vi "S2DS_INSTRUMENTS INVENTORY.vi"(5 "Instrument Info (in)":T2, 6 "Port list (in)":T1, 7 "error in":errorcluster) -> (0 "Instrument info (out)":T2, 1 "Port lists (out)":T1, 2 "OK 2":bool, 3 "Error (out)":errorcluster, 4 "Use array instrument":bool)   [LabVIEW 2025]
uses:
  TYPE DEFS/S2DS_VISA Read.ctl
  INST DRIVERS/My Current source/KE622x -- Output Low Connection.ctl
  INST DRIVERS/My Current source/KE622x -- Current Range.ctl
  INST DRIVERS/My Current source/KE622x -- Current Ranges.ctl
  TYPE DEFS/S2DS_Port lists.ctl
  TYPE DEFS/S2DS_Instrument Info.ctl
  TYPE DEFS/S2DS_Instrument parameters.ctl
  TYPE DEFS/S2DS_External write instrument settings.ctl
  INST DRIVERS/DAQ/MyDaq.lvlib
  INST DRIVERS/Cryo/Cryo.lvlib
  INST DRIVERS/DilutionFridge/MyTriton.lvlib
  INST DRIVERS/MySMU/MySMU.lvlib
  INST DRIVERS/My Current source/My Current Source.lvlib
panel:
  in  "Clear error":bool
  in  "Tab Control":T4(tab)
  in  "DAQ AO Address":tag[](array[tag]) caption="DAQ AO Addresses"
  in  "Min":dbl[](array[numeric])=[-10.0, -10.0, -10.0, -10.0]
  in  "Max":dbl[](array[numeric])=[10.0, 10.0, 10.0, 10.0]
  out "DAQ AO names":string[](array[string])=["DAQ1 AO 0", "DAQ1 AO 1", "DAQ2 AO 0", "DAQ2 AO 1"]
  out "DAQ  AI names":string[](array[string])=["DAQ1 AO 0", "DAQ1 AO 1", "DAQ2 AO 0", "DAQ2 AO 1"]
  in  "DAQ AI address":tag[](array[tag]) caption="DAQ AI Addresses"
  out "Present values":dbl[](array[numeric])
  in  "Use DAQ?":bool
  in  "Use Lock in 4":bool
  in  "Input ports 4":u16(ring) caption="Output ports" items=["None", "Sine out freq, amp", "AUX OUT", "Both Sine out and AUX OUT"]
  in  "Output ports 4":u16(ring) caption="Input ports" items=["X,Y,R,Theta", "Only AUX IN", "X,Y,R,Theta,AUX IN"]
  in  "VISA resource name lock in 4":refnum<visa-resource-name>
  in  "Measuring mode 4":enum16{"Voltage", "Current"}(ring) caption="Measuring mode"
  in  "Measuring mode 1":enum16{"Voltage", "Current"}(ring) caption="Measuring mode"
  in  "Use Lock in 1":bool
  in  "VISA resource name lock in 1":refnum<visa-resource-name>
  in  "Input ports":u16(ring) items=["X,Y,R,Theta", "Only AUX IN", "X,Y,R,Theta,AUX IN"]
  in  "Output ports":u16(ring)=1 items=["None", "Sine out freq, amp", "AUX OUT", "Both Sine out and AUX OUT"]
  in  "Use Lock in 2":bool
  in  "Input ports 2":u16(ring) caption="Output ports" items=["None", "Sine out freq, amp", "AUX OUT", "Both Sine out and AUX OUT"]
  in  "Output ports 2":u16(ring) caption="Input ports" items=["X,Y,R,Theta", "Only AUX IN", "X,Y,R,Theta,AUX IN"]
  in  "VISA resource name lock in 2":refnum<visa-resource-name>
  in  "Use Lock in 3":bool
  in  "Input ports 3":u16(ring) caption="Output ports" items=["None", "Sine out freq, amp", "AUX OUT", "Both Sine out and AUX OUT"]
  in  "Output ports 3":u16(ring) caption="Input ports" items=["X,Y,R,Theta", "Only AUX IN", "X,Y,R,Theta,AUX IN"]
  in  "VISA resource name lock in 3":refnum<visa-resource-name>
  in  "Measuring mode 2":enum16{"Voltage", "Current"}(ring)=enum."Current" caption="Measuring mode"
  in  "Measuring mode 3":enum16{"Voltage", "Current"}(ring) caption="Measuring mode"
  in  "Auto clear error? 2":bool caption="Auto clear error?"
  in  "Precision 2":dbl=0.0001 caption="Precision"
  in  "GPIB address":string="25"
  in  "Use wet cryo magnet?":bool
  in  "Select channel":u16(ring)=8 items=["PT2 Head"=1, "PT2 Plate"=2, "Still Plate"=3, "Cold Plate"=4, "MC Plate Cernox"=5, "PT1 Head"=6, "PT1 Plate"=7, "MC Plate RuO2"=8, "Magnet"=13]
  in  "Use DF?":bool caption="Use  Triton RI?"
  in  "Hold at end?":bool=TRUE
  in  "Precision":dbl=0.001
  in  "Auto clear error?":bool=TRUE
  in  "Initialize magnet?":bool
  in  "Initialize cryo magnet?":bool
  in  "Info magnet":bool
  in  "IP address":string="192.168.0.107"
  in  "Address":refnum<visa-resource-name>
  in  "Write Temp":string(combo)="03GPT"
  in  "Montana":bool caption="Lakeshore temperature controller"
  in  "Precesion":dbl
  in  "Timeout (s)":i32
  in  "TCP Address":string="10.0.0.3"
  in  "Wait time (s)":i32
  in  "Read  Temp":string(combo)="03GPT"
  in  "Timeout (s)":i32=60
  in  "Wait time (s)":i32=30
  in  "Precesion (K)":dbl=0.05
  in  "Lakeshore 336":bool caption="Lakeshore temperature controller"
  in  "Ramp":bool=TRUE
  in  "Ramp rate (K/min)":dbl=1.0
  in  "Resset SMU? 2":bool
  in  "Source Value":dbl
  in  "Compliance Limit":dbl
  in  "Source":u16(ring)=1 items=["Current", "Voltage"]
  in  "Use SMU?":bool caption="DS360 Function generator"
  in  "SMU VISA Address":refnum<visa-resource-name>
  in  "Measure":u16(ring) items=["Current", "Voltage"]
  in  "Use Current source?":bool caption="DS360 Function generator"
  in  "Current source VISA Address":refnum<visa-resource-name>
  in  "Current level":dbl format="%#_13g"
  in  "Current Range In":T5={"Auto Range?"=TRUE, "Man / Selected\nRange"=enum."2nA"}
  in  "Resset SMU?":bool
  in  "Output Low \nConnection":T7
  in  "Voltage limit (V)":dbl format="%#_13g"
  in  "Use Keithley 2182 Nanovoltmeter?":bool caption="DS360 Function generator"
  in  "Keithley 2182 address":refnum<visa-resource-name>
  in  "Lakeshore temperature controller GPIB address":refnum<visa-resource-name>="12"
  in  "Use Lakeshore?":bool caption="Lakeshore temperature controller"
  in  "DS360 Function Generator GPIB address":string="8"
  in  "Use DS360 Func Gen?":bool caption="DS360 Function generator"
  in  "Use ITC He3?":bool caption="Lakeshore temperature controller"
  in  "VISA Address":refnum<visa-resource-name> caption="ITC 503"
  in  "Read Item":u16(ring)=1 items=["Setpoint", "Sensor 1", "Sensor 2", "Sensor 3", "Temperature Error", "Heater Output (%)", "Heater Output (V)", "Gas Flow Output", "P Term", "I term", "D term", "Channel 1 Frequency/4", "Channel 2 Frequency/4", "Channel 3 Frequency/4"]
  in  "Use AH2700A?":bool caption="Lakeshore temperature controller"
  in  "VISA Address 2":refnum<visa-resource-name> caption="AH2700A Capacitance Bridge"
  in  "Initialize AH2700A?":bool
  in  "TEST GR1 4":bool
  in  "TEST GR1 3":bool
  in  "TEST GR1 2":bool
  in  "TEST GR1":bool
  in  "Visa Read":T8={"VISA resource"="", "Read Command"="", "Format string"="%f "}
  in  "Use VISA Read 1":bool caption="GPIB read 1"
  in  "TEST GW1":bool
  in  "GW1 String 1":string
  in  "Use  GPIB Write 1?":bool caption="GW1"
  in  "VISA resource name GW1":refnum<visa-resource-name>
  in  "Use  GPIB Write 4?":bool caption="GW4"
  in  "GW4 String 2":string
  in  "VISA resource name GW4":refnum<visa-resource-name>
  in  "TEST GW4":bool
  in  "Use  GPIB Write 2?":bool caption="GW2"
  in  "GW2 String 1":string
  in  "VISA resource name GW2":refnum<visa-resource-name>
  in  "TEST GW1 2":bool
  in  "Use  GPIB Write 3?":bool caption="GW3"
  in  "GW3 String 1":string
  in  "VISA resource name GW3":refnum<visa-resource-name>
  in  "TEST GW1 3":bool
  in  "Use VISA Read 2":bool caption="GPIB read 1"
  in  "Visa Read 2":T8={"VISA resource"="", "Read Command"="", "Format string"="%f "} caption="Visa Read"
  in  "Visa Read 3":T8={"VISA resource"="", "Read Command"="", "Format string"="%f "} caption="Visa Read"
  in  "Use VISA Read 3":bool caption="GPIB read 1"
  in  "Visa Read 4":T8={"VISA resource"="", "Read Command"="", "Format string"="%f "} caption="Visa Read"
  in  "Use VISA Read 4":bool caption="GPIB read 1"
  in  "Use External 2?":bool caption="DS360 Function generator"
  in  "?":T9={"Check for response?"=FALSE, "Pooling time out (ms)"=100, "Precision"=1e-06, "IP"="localhost"}
  in  "Use External 1?":bool caption="DS360 Function generator"
  in  "?":T9={"Check for response?"=FALSE, "Pooling time out (ms)"=100, "Precision"=1e-06, "IP"="localhost"}
  in  "Use array instrument":bool caption="DS360 Function generator"
  out "Error status:":errorcluster
  in  "OK":bool
  # "Instrument inventory..."
  # "Before accepting:\n 1. Check all required ports\n 2. Uncheck the others\n 3. Ensure no error"
  # "Lock In 2"
  # "Lock In 1"
  # "Lock In 3"
  # "Lock In 4"
  # "Magnet"
  # "Temperature"
  # "Command format"
  # "Address"
  # "Command"
  # "Format string"
  # "Test"
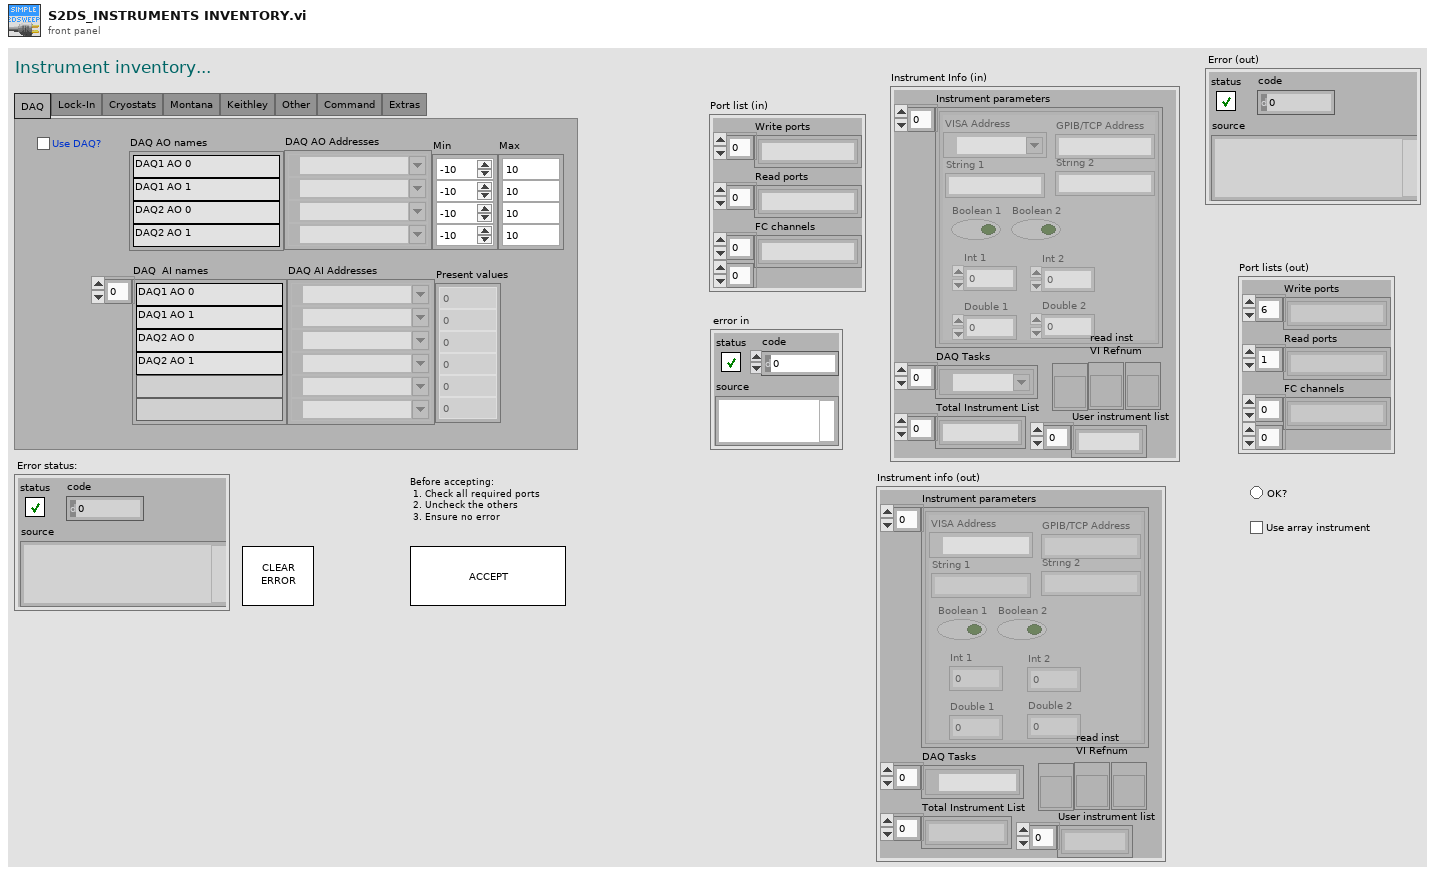
[diagram p1: front panel]
types:
  T1 = typedef "S2DS_Port lists.ctl" = cluster{"Write ports":string[], "Read ports":string[], "FC channels":string[][]}
  T2 = typedef "S2DS_Instrument Info.ctl" = cluster{"Instrument parameters":T3[], "DAQ Tasks":refnum<k21>[], "Total Instrument List":string[], "read inst \nVI Refnum":refnum<vi>, "type specifier Edit instruments VI Refnum":refnum<vi>, "type specifier write instrument VI Refnum (for type only)":refnum<vi>, "User instrument list":string[]}
  T3 = typedef "S2DS_Instrument parameters.ctl" = cluster{"VISA Address":refnum<visa-resource-name>, "GPIB/TCP Address":string, "String 1":string, "String 2":string, "Boolean 1":bool, "Boolean 2":bool, "Int 1":i32, "Int 2":i32, "Double 1":dbl, "Double 2":dbl}
  T4 = enum32{"DAQ", "Lock-In", "Cryostats", "Montana", "Keithley", "Other", "Command", "Extras"}
  T5 = typedef "My Current Source.lvlib/KE622x -- Current Range.ctl" = cluster{"Auto Range?":bool, "Man / Selected\nRange":T6}
  T6 = typedef "My Current Source.lvlib/KE622x -- Current Ranges.ctl" = enum16{"2nA", "20nA", "200nA", "2uA", "20uA", "200uA", "2mA", "20mA", "100mA"}
  T7 = typedef "My Current Source.lvlib/KE622x -- Output Low Connection.ctl" = enum16{"Floating", "Earth Ground"}
  T8 = typedef "S2DS_VISA Read.ctl" = cluster{"VISA resource":refnum<visa-resource-name>, "Read Command":string, "Format string":string}
  T9 = typedef "S2DS_External write instrument settings.ctl" = cluster{"Check for response?":bool, "Pooling time out (ms)":i32, "Precision":dbl, "IP":string}
  T10 = cluster{"VISA Address":refnum<visa-resource-name>, "GPIB/TCP Address":string, "String 1":string, "String 2":string, "Boolean 1":bool, "Boolean 2":bool, "Integer 1":i32, "Integer 2":i32, "Double 1":dbl, "Double 2":dbl}
  T11 = cluster{"VISA Address":refnum<visa-resource-name>, "GPIB/TCP Address":string, "String 1":string, "String 2":string, "Boolean 1":bool, "Boolean 2":bool, "Integer 1":i32, "Integer 2":i32, "Double 1":dbl, "Double 2":dbl}[]
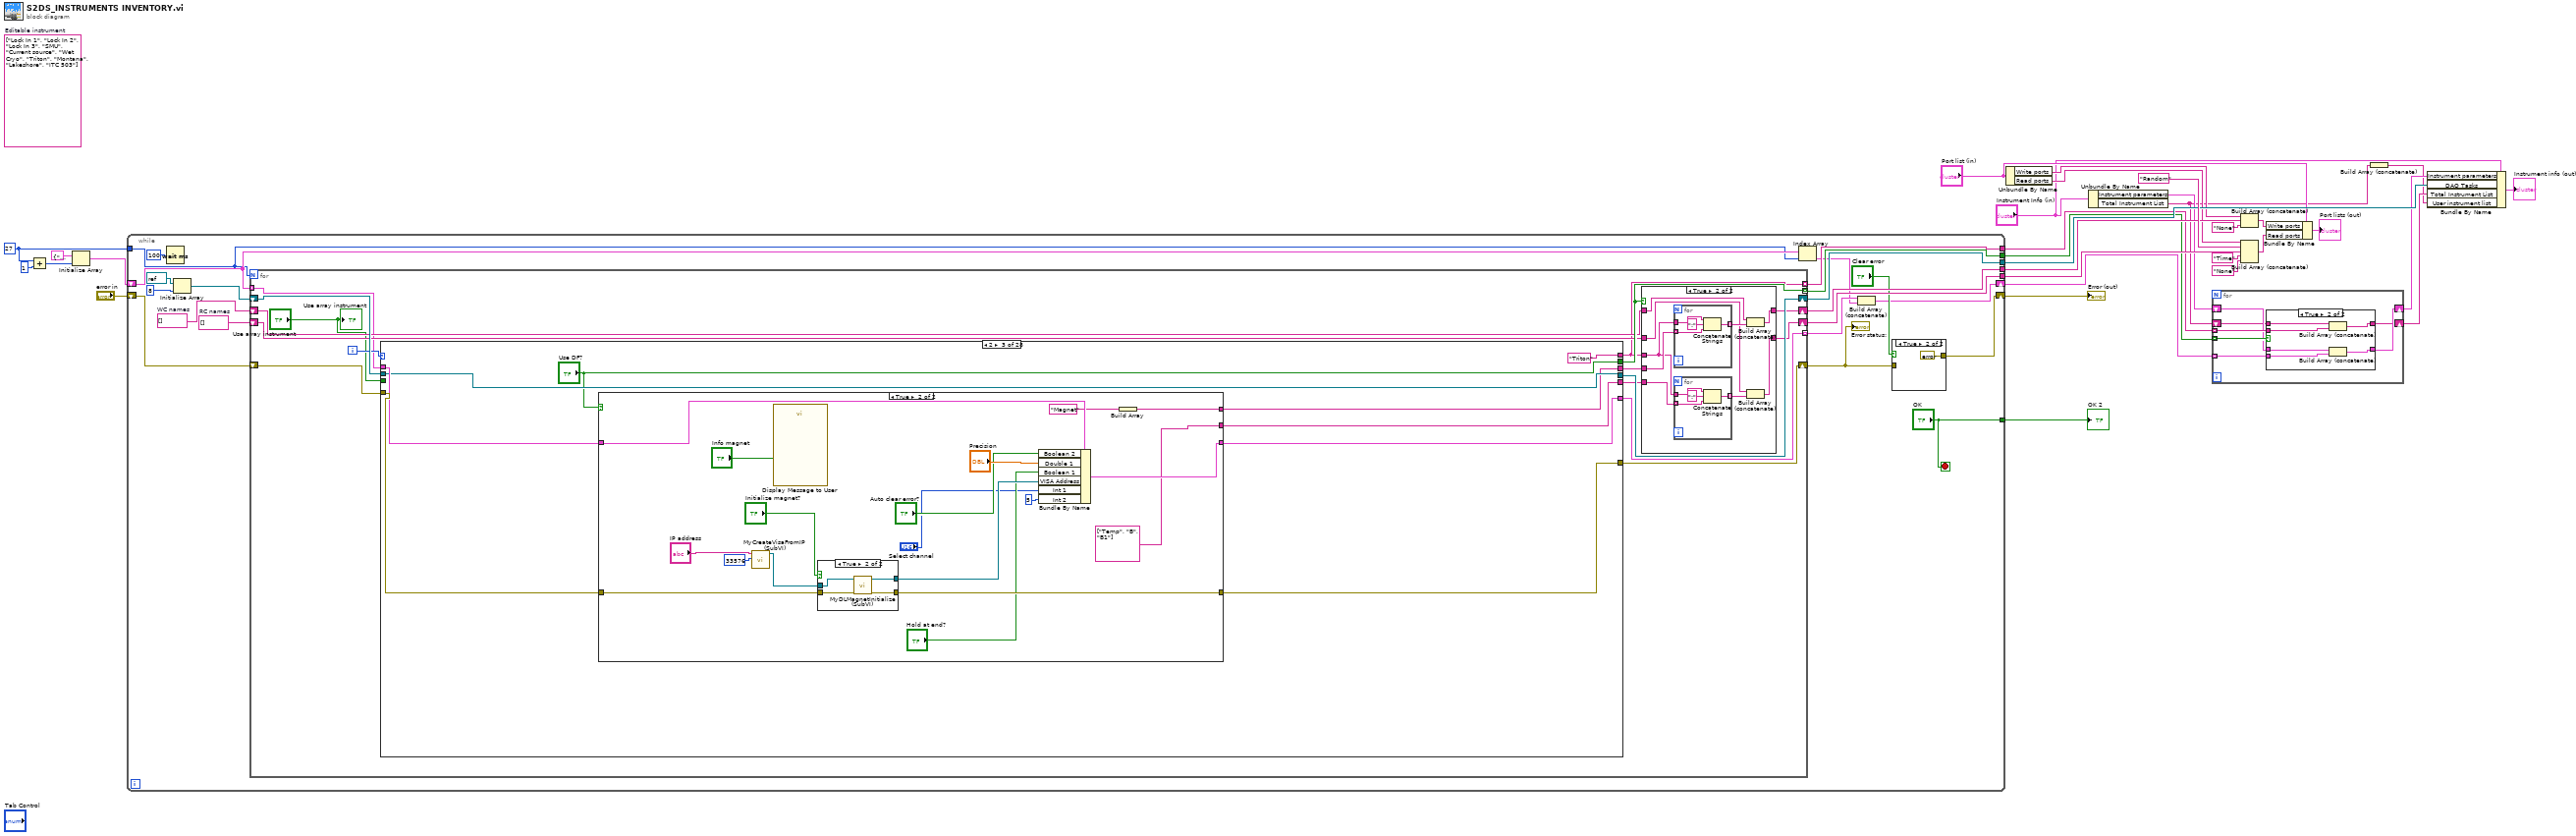
[diagram p0: block diagram]
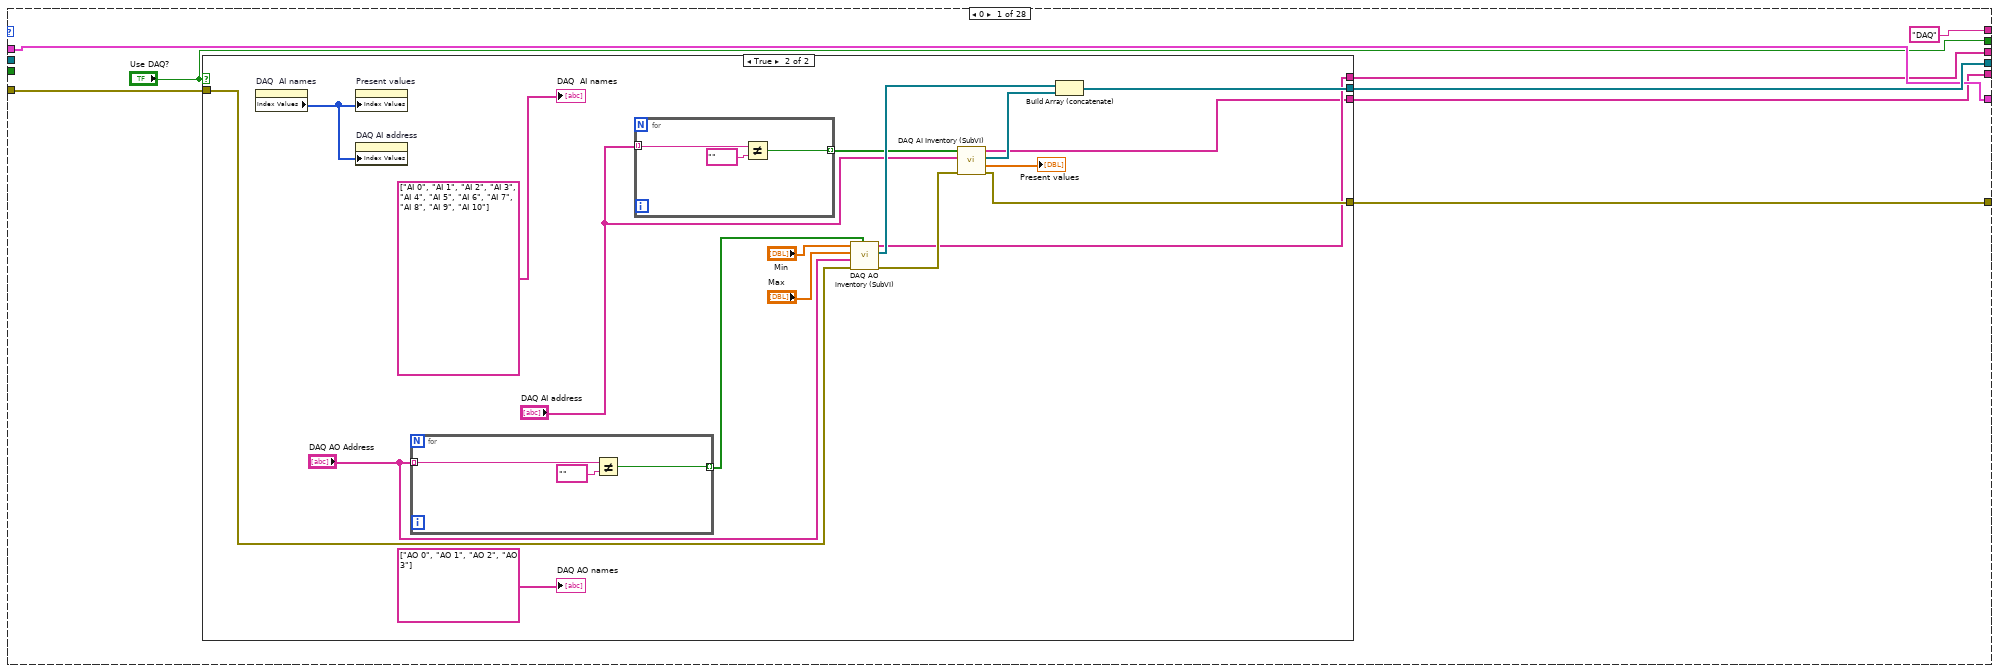
[diagram p5: hidden frame]
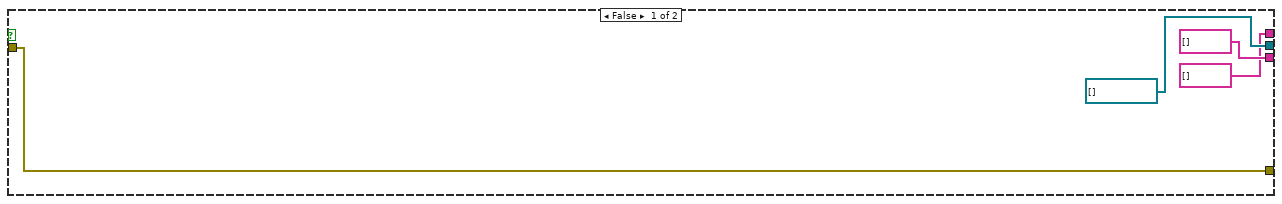
[diagram p6: hidden frame]
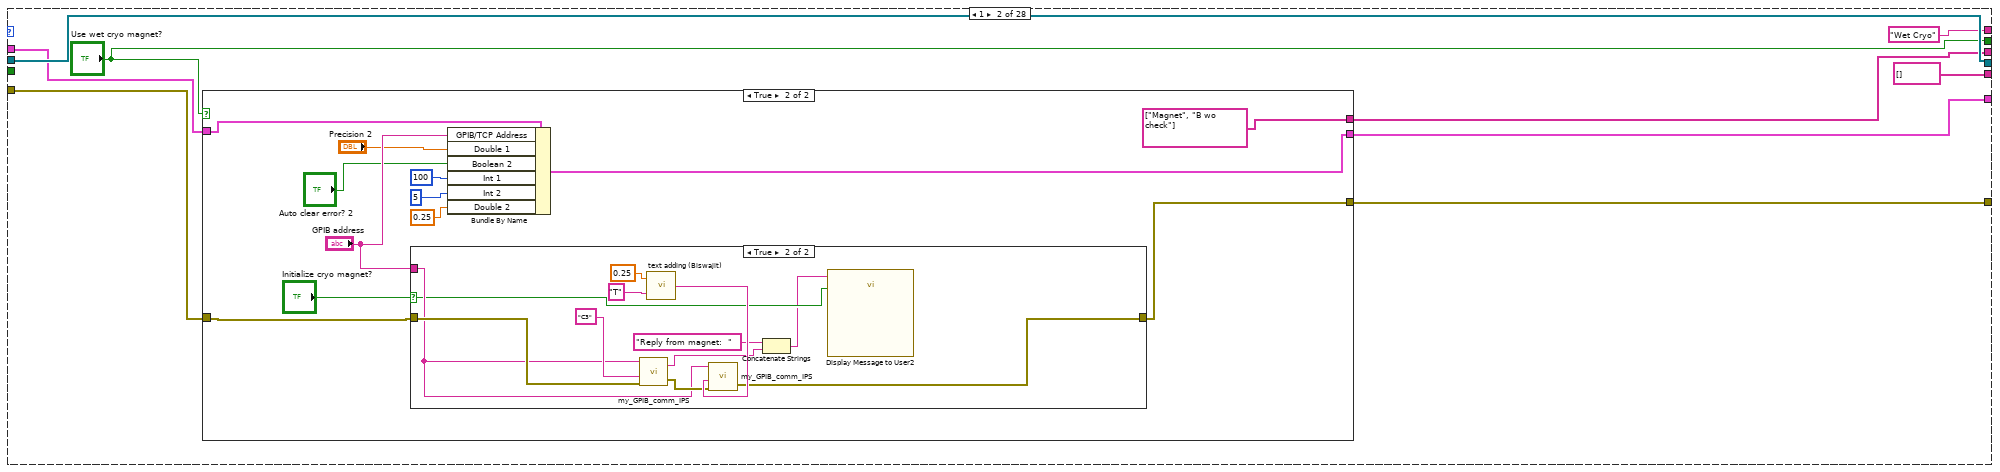
[diagram p7: hidden frame]
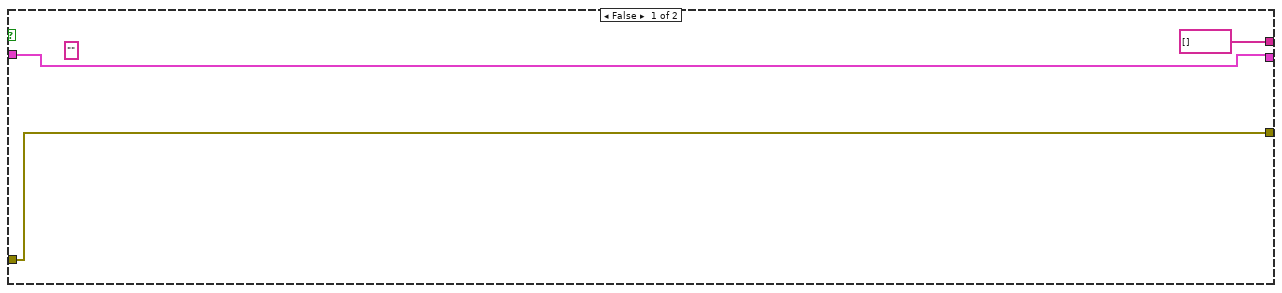
[diagram p8: hidden frame]
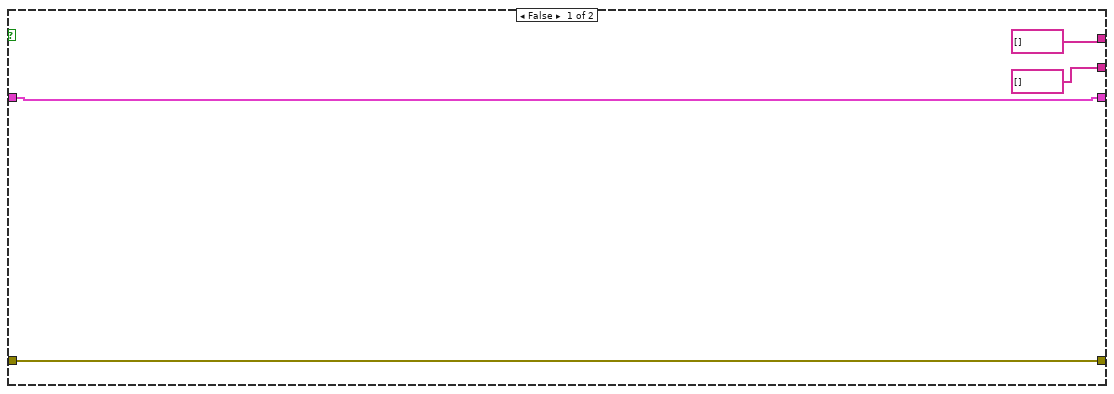
[diagram p10: hidden frame]
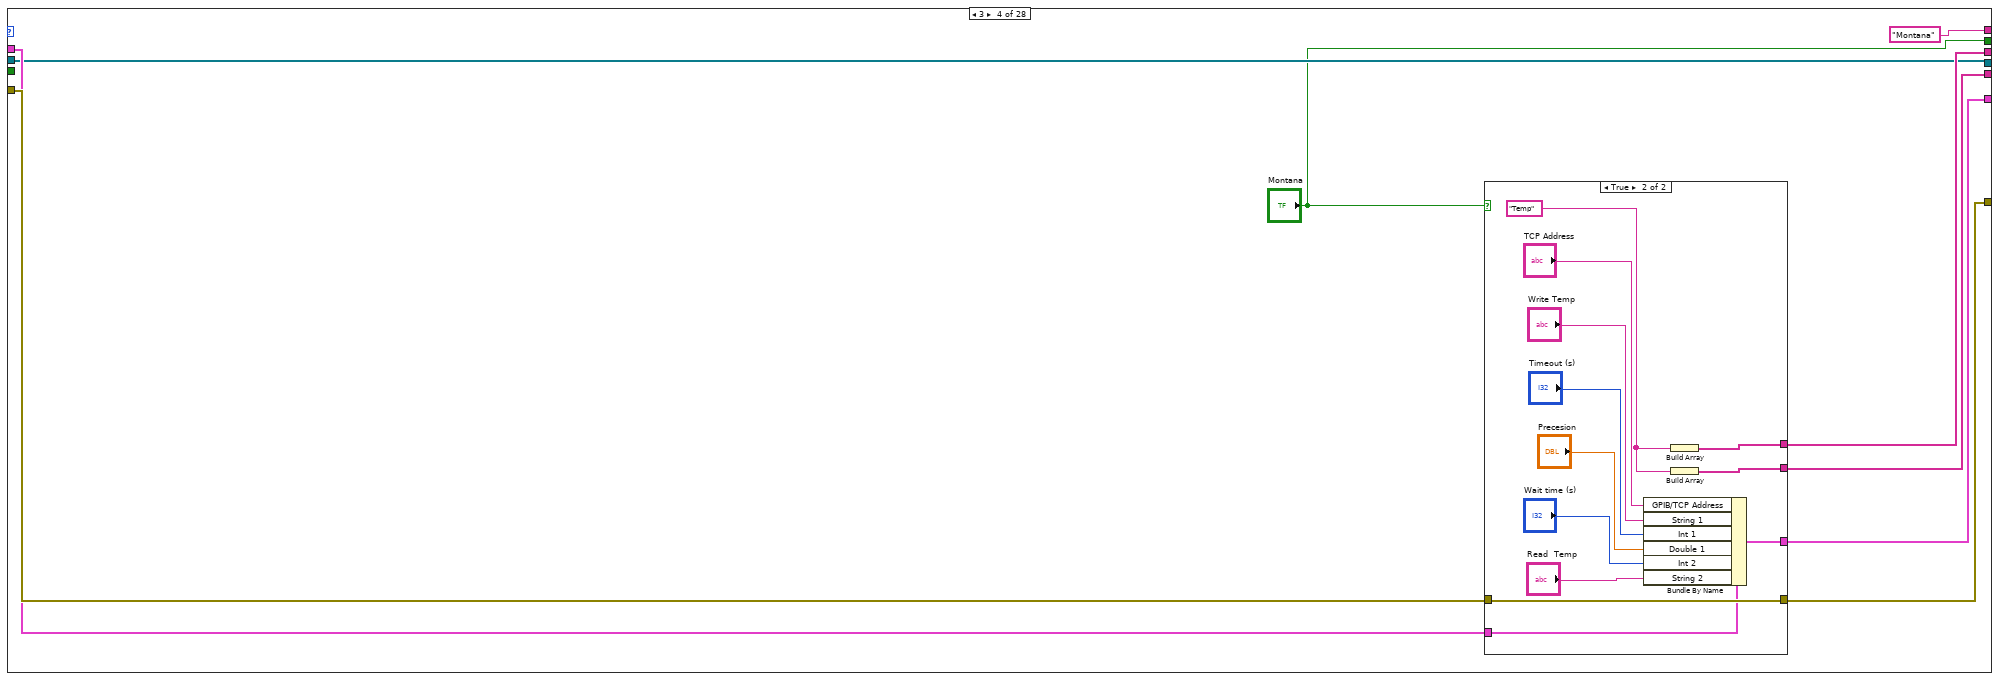
[diagram p12: hidden frame]
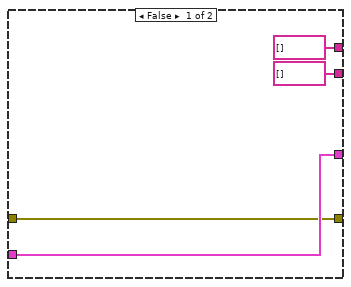
[diagram p13: hidden frame]
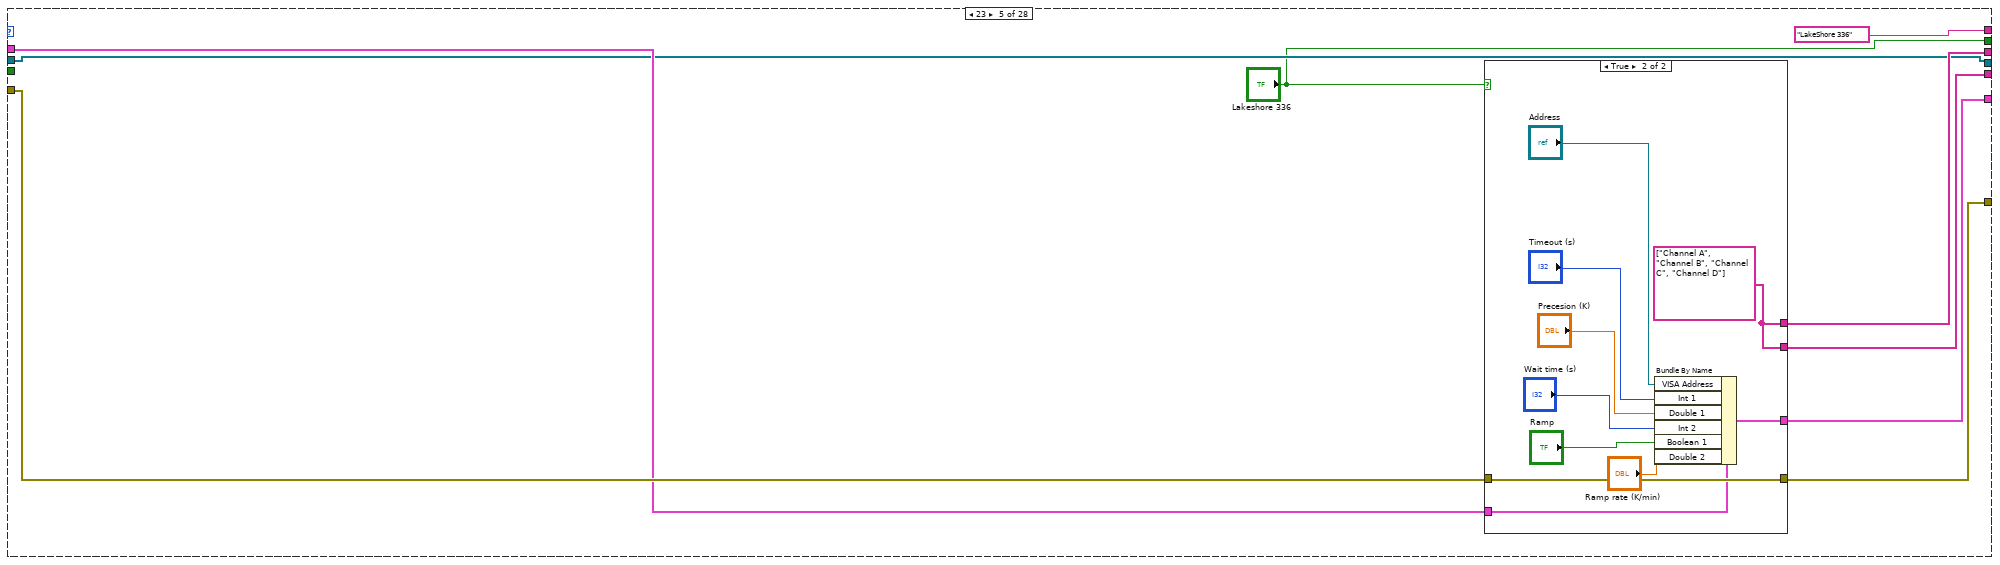
[diagram p14: hidden frame]
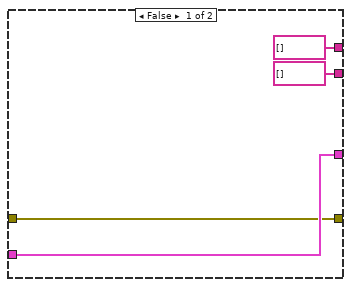
[diagram p15: hidden frame]
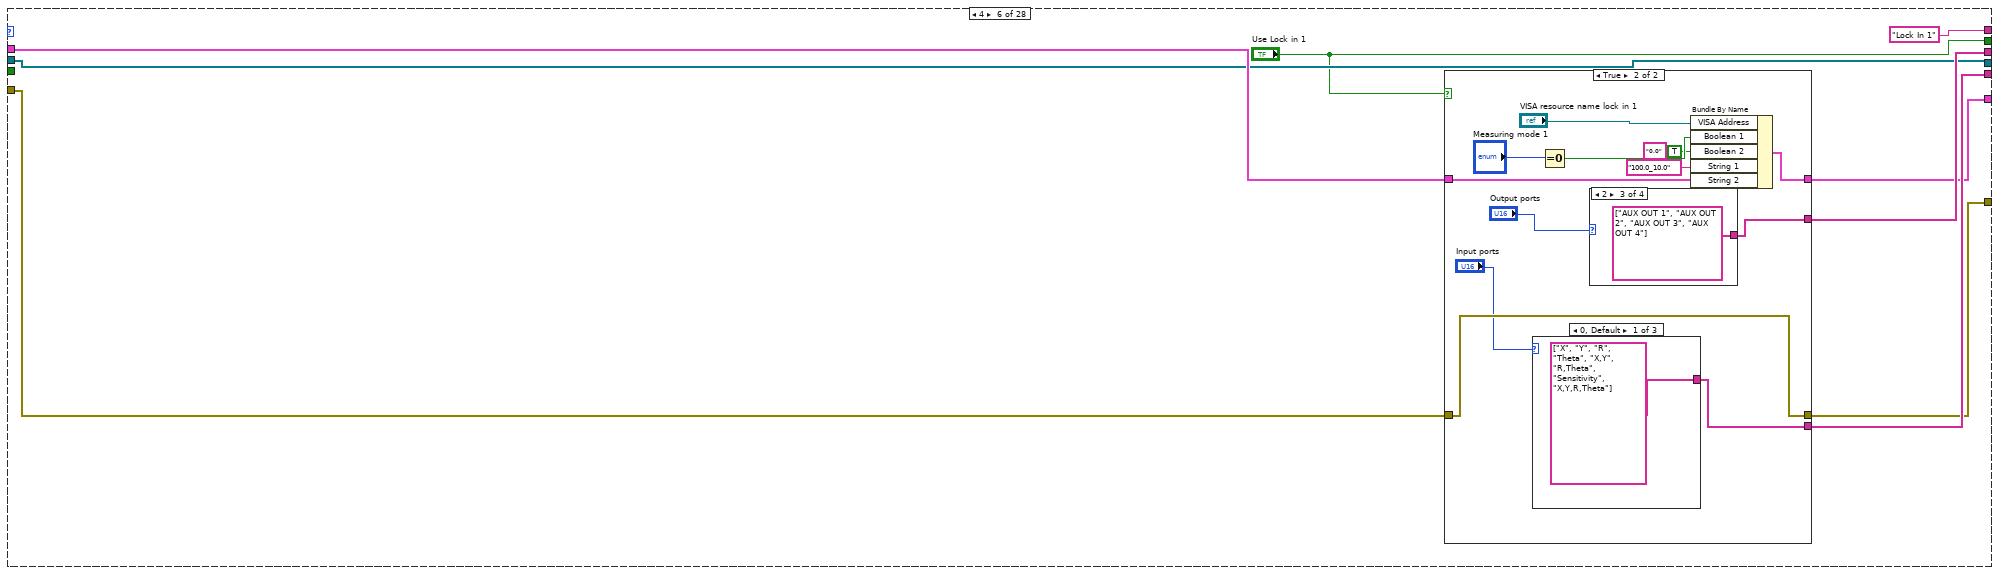
[diagram p16: hidden frame]
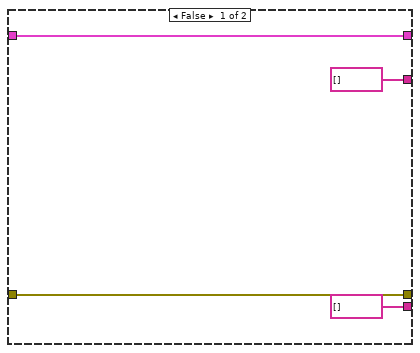
[diagram p17: hidden frame]
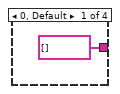
[diagram p18: hidden frame]
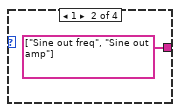
[diagram p19: hidden frame]
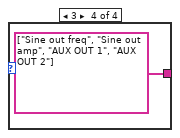
[diagram p20: hidden frame]
diagram:
  w7 = 27
  (unwired) string[] ["Lock In 1", "Lock In 2", "Lock In 3", "SMU", "Current source", "Wet Cryo", "Triton", "Montana", "Lakeshore", "ITC 503"]  # Editable instrument
  n1 = Add(x=w7, y=1 ("index")) -> (x+y=w5:i32)
  n2 = Initialize Array(T10 {"VISA Address"="", "GPIB/TCP Address"="", "String 1"="", "String 2"="", "Boolean 1"=FALSE, "Boolean 2"=FALSE, "Integer 1"=0, "Integer 2"=0, "Double 1"=0.0, "Double 2"=0.0} ("Instrument parameters"), w5) -> (w13:T11)
  n3 = while {
    tunnel: [w48] -> w23
    tunnel: [w46] -> w31
    tunnel: [w47] -> w29
    shift-right: [w40] -> w16
    shift-left: "error in" -> [w42]
    shift-right: [w36] -> w11
    shift-left: w13 -> [w34]
    tunnel: [w39] -> w12
    tunnel: [w38] -> w3
    tunnel: w7 -> [w33]
    tunnel: ["OK"] -> w4
    stop <- "OK" stop-if-true
    w45 = string[] []  # RC names
    w44 = string[] []  # WC names
    n4 = Wait (ms)(milliseconds to wait=u32 100) -> ()  [unwired: 1 out]
    n5 = Initialize Array(refnum<k21> refnum ("task out"), 8 ("dimension size")) -> (w49:refnum<k21>[])
    n6 = for {
      N: w33 -> [_]
      shift-right: [w70] -> w43
      shift-left: w42 -> [w58]
      shift-right: [w63] -> w46
      shift-left: w45 -> [w64]
      shift-right: [w65] -> w47
      shift-left: w44 -> [w66]
      shift-right: [w68] -> w48
      shift-left: w49 -> [w69]
      tunnel: [w67] -> w39 mode=indexing
      tunnel: w34 -> [w61] mode=indexing
      tunnel: [w60] -> w37 mode=indexing
      tunnel: [w59] -> w38 mode=indexing
      i -> [w62]
      n7 = case shown="2" w62 {
        tunnel: w58 -> [w97 w134 w171 w207 w232 w256 w289 w322 w355 w387 w404 w424 w451 w479 w507 w535 w562 w587 w612 w637 w663 w690 w707 w730 w758 w778 w798 w815]
        tunnel: [w95 w133 w168 w208 w233 w252 w285 w318 w351 w386 w403 w423 w448 w476 w504 w533 w560 w585 w610 w635 w661 w688 w705 w728 w756 w776 w796 w815] -> w70
        tunnel: [w92 w130 w167 w204 w229 w254 w287 w320 w353 string[] [] ("RC names") string[] [] ("RC names") string[] [] ("RC names") w447 w475 w503 w532 string[] [] ("RC names") string[] [] ("RC names") string[] [] ("RC names") string[] [] ("RC names") w659 w684 w701 w725 w753 w773 w793 w813] -> w57
        tunnel: [w91 string[] [] ("RC names") w163 w205 w230 w253 w286 w319 w352 w380 w397 w417 string[] [] ("RC names") string[] [] ("RC names") string[] [] ("RC names") string[] [] ("RC names") w559 w584 w609 w634 w660 string[] [] ("RC names") string[] [] ("RC names") w723 w751 w771 w792 w813] -> w56
        tunnel: w69 -> [_ w132 w169 w203 w228 w251 w284 w317 w350 w385 w402 w422 w449 w477 w505 w531 w561 w586 w611 w636 w658 w689 w706 w729 w757 w777 w797 w816]
        tunnel: [w96 w132 w169 w203 w228 w251 w284 w317 w350 w385 w402 w422 w449 w477 w505 w531 w561 w586 w611 w636 w658 w689 w706 w729 w757 w777 w797 w816] -> w68
        tunnel: w61 -> [w94 w131 w170 w206 w231 w255 w288 w321 w354 w388 w405 w425 w450 w478 w506 w534 w563 w588 w613 w638 w662 w691 w708 w731 w759 w779 w799 w814]
        tunnel: [w94 w128 w164 w202 w227 w250 w283 w316 w349 w384 w401 w421 w445 w473 w501 w529 w557 w582 w607 w632 w657 w687 w704 w727 w755 w775 w795 w814] -> w60
        tunnel: ["DAQ" "Wet Cryo" "Triton" "Montana" "LakeShore 336" "Lock In 1" "Lock In 2" "Lock In 3" "Lock In 4" "Lakeshore" "ITC 503" "AH2700A" "GW1" "GW2" "GW3" "GW4" "VISA Read 1" "VISA Read 2" "VISA Read 3" "VISA Read 4" "SMU" "DS360 FG" "Current source" "Keithley 2182" "External 1" "External 2" "Array" "d"] -> w59
        tunnel: ["Use DAQ?" "Use wet cryo magnet?" "Use DF?" "Montana" "Lakeshore 336" "Use Lock in 1" "Use Lock in 2" "Use Lock in 3" "Use Lock in 4" "Use Lakeshore?" "Use ITC He3?" "Use AH2700A?" "Use  GPIB Write 1?" "Use  GPIB Write 2?" "Use  GPIB Write 3?" "Use  GPIB Write 4?" "Use VISA Read 1" "Use VISA Read 2" "Use VISA Read 3" "Use VISA Read 4" "Use SMU?" "Use DS360 Func Gen?" "Use Current source?" "Use Keithley 2182 Nanovoltmeter?" "Use External 1?" "Use External 2?" w791 FALSE ("Use  GPIB Write 4?")] -> w67
        tunnel: "Use array instrument" -> [_ _ _ _ _ _ _ _ _ _ _ _ _ _ _ _ _ _ _ _ _ _ _ _ _ _ w791 _]
        frame 0 {
          n8 = case shown="True" "Use DAQ?" {
            tunnel: w97 -> [w101 w119]
            tunnel: [refnum<k21>[] [] w112] -> w96
            tunnel: [w101 w110] -> w95
            tunnel: [string[] [] ("DAQ names out") w109] -> w92
            tunnel: [string[] [] ("DAQ names out") w108] -> w91
            frame False {
            }
            frame True {
              n9 = property on="DAQ  AI names" class="Arr (strict)"() -> ("Index Values"=w102:u32[])  [unwired: 2 in, 2 out]
              n10 = property on="Present values" class="Arr (strict)"("Index Values"=w102) -> ()  [unwired: 2 in, 2 out]
              n11 = property on="DAQ AI address" class="Arr (strict)"("Index Values"=w102) -> ()  [unwired: 2 in, 2 out]
              n12 = for {
                tunnel: "DAQ AO Address" -> [w122] mode=indexing
                tunnel: [w120] -> w103 mode=indexing
                n13 = Not Equal?(x=w122, y=tag "") -> (x != y?=w120:bool)
              }
              n14 = for {
                tunnel: "DAQ AI address" -> [w125] mode=indexing
                tunnel: [w123] -> w105 mode=indexing
                n15 = Not Equal?(x=w125, y=tag "") -> (x != y?=w123:bool)
              }
              n16 = call "DAQ AO inventory (SubVI).vi"("Use DAQ AO?"=w103, "error in (no error)"=w119, "Address in"="DAQ AO Address", "Max"="Max", "Min"="Min") -> ("error out"=w111:errorcluster, "Address out"=w114:refnum<k21>[], "DAQ names out"=w109:string[])  [unwired: 4 in]
              n17 = call "DAQ AI Inventory (SubVI).vi"("error in (no error)"=w111, "DAQ AI address"="DAQ AI address", "Use DAQ AI?"=w105) -> ("error out"=w110:errorcluster, "present values out"=→"Present values":dbl[], "DAQ AI Address out"=w113:refnum<k21>[], "DAQ names out"=w108:string[])  [unwired: 5 in]
              n18 = Build Array (concatenate)(w114, w113) -> (w112:refnum<k21>[])
              "DAQ AO names" <- string[] ["AO 0", "AO 1", "AO 2", "AO 3"] ("Array 2")
              "DAQ  AI names" <- string[] ["AI 0", "AI 1", "AI 2", "AI 3", "AI 4", "AI 5", "AI 6", "AI 7", "AI 8", "AI 9", "AI 10"] ("Array 2")
            }
          }
        }
        frame 1 {
          n19 = case shown="True" "Use wet cryo magnet?" {
            tunnel: w134 -> [w137 w149]
            tunnel: [w137 w148] -> w133
            tunnel: [string[] [] string[] ["Magnet", "B wo check"]] -> w130
            tunnel: w131 -> [w136 w147]
            tunnel: [w136 w145] -> w128
            frame False {
              (unwired) "" ("IPS GPIB address")
            }
            frame True {
              n20 = case shown="True" "Initialize cryo magnet?" {
                selector: "Initialize cryo magnet?" -> [_ w154]
                tunnel: w149 -> [w150 w158]
                tunnel: [w150 w156] -> w148
                tunnel: "GPIB address" -> [_ w155]
                frame False {
                }
                frame True {
                  n21 = call "my_GPIB_comm_IPS.vi"("error in"=w158, "Command"="C3", "GPIB address"=w155) -> ("error out"=w157:errorcluster, "Reply from Instrument"=w153:string)  [unwired: 1 in]
                  n22 = call "text adding (Biswajit).vi"("string"="T", "number"=0.25 ("Sweep rate (T/min)")) -> ("String"=w161:string)
                  n23 = call "my_GPIB_comm_IPS.vi"("error in"=w157, "Command"=w161, "GPIB address"=w155) -> ("error out"=w156:errorcluster)  [unwired: 1 in, 1 out]
                  n24 = Concatenate Strings("Reply from magnet:  " ("string"), w153) -> (w152:string)
                  n25 = call "Display Message to User2"("Enable"=w154, "Message"=w152) -> ()  [unwired: 8 in, 2 out]
                }
              }
              n26 = Bundle By Name(cluster=w147, "GPIB/TCP Address"="GPIB address", "Double 1"="Precision 2", "Boolean 2"="Auto clear error? 2", "Int 1"=100, "Int 2"=5, "Double 2"=0.25) -> (w145:T3)
            }
          }
        }
        frame 2 {
          n27 = case shown="True" "Use DF?" {
            tunnel: w170 -> [w175 w193]
            tunnel: [w175 w192] -> w164
            tunnel: [string[] [] w190] -> w167
            tunnel: [w174 w188] -> w168
            tunnel: w171 -> [w174 w189]
            tunnel: [string[] [] string[] ["Temp", "B", "B1"]] -> w163
            frame False {
            }
            frame True {
              n28 = call "MyCreateVisaFromIP (SubVI).vi"("Port"=33576, "IP address"="IP address") -> ("VISA Refnum out"=w179:refnum<visa-resource-name>)  [unwired: 9 in]
              n29 = call "Display Message to User"("Enable"="Info magnet") -> ()  [unwired: 9 in, 2 out]
              n30 = case shown="True" "Initialize magnet?" {
                tunnel: w179 -> [w194 w199]
                tunnel: w189 -> [w195 w198]
                tunnel: [w195 w197] -> w188
                tunnel: [w194 w196] -> w187
                frame False {
                }
                frame True {
                  n31 = call "MyDLMagnetInitialize (SubVI).vi"("error in"=w198, "VISA resource name in"=w199) -> ("error out"=w197:errorcluster, "VISA Refnum out"=w196:refnum<visa-resource-name>)  [unwired: 8 in]
                }
              }
              n32 = Bundle By Name(cluster=w193, "Boolean 2"="Auto clear error?", "Double 1"="Precision", "Boolean 1"="Hold at end?", "VISA Address"=w187, "Int 1"="Select channel", "Int 2"=5) -> (w192:T3)
              n33 = Build Array("Magnet") -> (w190:string[])
            }
          }
        }
        frame 3 {
          n34 = case shown="True" "Montana" {
            tunnel: [string[] [] w224] -> w205
            tunnel: w206 -> [w212 w222]
            tunnel: [w212 w221] -> w202
            tunnel: w207 -> [w211 w223]
            tunnel: [w211 w223] -> w208
            tunnel: [string[] [] w215] -> w204
            frame False {
            }
            frame True {
              w214 = "Temp"
              n35 = Bundle By Name(cluster=w222, "GPIB/TCP Address"="TCP Address", "String 1"="Write Temp", "Int 1"="Timeout (s)", "Double 1"="Precesion", "Int 2"="Wait time (s)", "String 2"="Read  Temp") -> (w221:T3)
              n36 = Build Array(w214) -> (w215:string[])
              n37 = Build Array(w214) -> (w224:string[])
            }
          }
        }
        frame 23 {
          n38 = case shown="True" "Lakeshore 336" {
            tunnel: [string[] [] w240] -> w230
            tunnel: w231 -> [w237 w246]
            tunnel: [w237 w245] -> w227
            tunnel: w232 -> [w236 w247]
            tunnel: [w236 w247] -> w233
            tunnel: [string[] [] w240] -> w229
            frame False {
            }
            frame True {
              w240 = string[] ["Channel A", "Channel B", "Channel C", "Channel D"]
              n39 = Bundle By Name(cluster=w246, "VISA Address"="Address", "Int 1"="Timeout (s)", "Double 1"="Precesion (K)", "Int 2"="Wait time (s)", "Boolean 1"="Ramp", "Double 2"="Ramp rate (K/min)") -> (w245:T3)
            }
          }
        }
        frame 4 {
          n40 = case shown="True" "Use Lock in 1" {
            tunnel: w256 -> [w260 w270]
            tunnel: [w260 w270] -> w252
            tunnel: [string[] [] w266] -> w253
            tunnel: [string[] [] w269] -> w254
            tunnel: w255 -> [w259 w273]
            tunnel: [w259 w271] -> w250
            frame False {
            }
            frame True {
              n41 = case shown="0, Default" "Input ports" {
                tunnel: [string[] ["X", "Y", "R", "Theta", "X,Y", "R,Theta", "Sensitivity", "X,Y,R,Theta"] string[] ["AUX IN 1", "AUX IN 2", "AUX IN 3", "AUX IN 4"] string[] ["X", "Y", "R", "Theta", "AUX IIN 1", "AUX IN 2", "Sensitivity", "X,Y", "R,Theta"]] -> w266
                frame 0, Default {
                }
                frame 1 {
                }
                frame 2 {
                }
              }
              n42 = Equal To 0?(x="Measuring mode 1") -> (x = 0?=w264:bool)
              n43 = case shown="2" "Output ports" {
                tunnel: [string[] [] ("Array") string[] ["Sine out freq", "Sine out amp"] ("Array") string[] ["AUX OUT 1", "AUX OUT 2", "AUX OUT 3", "AUX OUT 4"] ("Array") string[] ["Sine out freq", "Sine out amp", "AUX OUT 1", "AUX OUT 2"] ("Array")] -> w269
                frame 0, Default {
                }
                frame 1 {
                }
                frame 2 {
                }
                frame 3 {
                }
              }
              n44 = Bundle By Name(cluster=w273, "VISA Address"="VISA resource name lock in 1", "Boolean 1"=w264, "Boolean 2"=TRUE, "String 1"="100.0_10.0", "String 2"="0.0") -> (w271:T3)
            }
          }
        }
        frame 5 {
          n45 = case shown="True" "Use Lock in 2" {
            tunnel: w289 -> [w293 w303]
            tunnel: [w293 w303] -> w285
            tunnel: [string[] [] w294] -> w286
            tunnel: [string[] [] w302] -> w287
            tunnel: w288 -> [w292 w306]
            tunnel: [w292 w304] -> w283
            frame False {
            }
            frame True {
              n46 = case shown="0, Default" "Output ports 2" {
                tunnel: [string[] ["X", "Y", "R", "Theta", "X,Y", "R,Theta", "Sensitivity", "X,Y,R,Theta"] string[] ["AUX IN 1", "AUX IN 2", "AUX IN 3", "AUX IN 4"] string[] ["X", "Y", "R", "Theta", "AUX IIN 1", "AUX IN 2", "Sensitivity", "X,Y", "R,Theta"]] -> w294
                frame 0, Default {
                }
                frame 1 {
                }
                frame 2 {
                }
              }
              n47 = Equal To 0?(x="Measuring mode 2") -> (x = 0?=w299:bool)
              n48 = case shown="2" "Input ports 2" {
                tunnel: [string[] [] ("Array") string[] ["Sine out freq", "Sine out amp"] ("Array") string[] ["AUX OUT 1", "AUX OUT 2", "AUX OUT 3", "AUX OUT 4"] ("Array") string[] ["Sine out freq", "Sine out amp", "AUX OUT 1", "AUX OUT 2"] ("Array")] -> w302
                frame 0, Default {
                }
                frame 1 {
                }
                frame 2 {
                }
                frame 3 {
                }
              }
              n49 = Bundle By Name(cluster=w306, "VISA Address"="VISA resource name lock in 2", "Boolean 1"=w299, "Boolean 2"=TRUE, "String 1"="100.0_10.0", "String 2"="0.0") -> (w304:T3)
            }
          }
        }
        frame 6 {
          n50 = case shown="True" "Use Lock in 3" {
            tunnel: w322 -> [w326 w336]
            tunnel: [w326 w336] -> w318
            tunnel: [string[] [] w327] -> w319
            tunnel: [string[] [] w335] -> w320
            tunnel: w321 -> [w325 w339]
            tunnel: [w325 w337] -> w316
            frame False {
            }
            frame True {
              n51 = case shown="0, Default" "Output ports 3" {
                tunnel: [string[] ["X", "Y", "R", "Theta", "X,Y", "R,Theta", "Sensitivity", "X,Y,R,Theta"] string[] ["AUX IN 1", "AUX IN 2", "AUX IN 3", "AUX IN 4"] string[] ["X", "Y", "R", "Theta", "AUX IIN 1", "AUX IN 2", "Sensitivity", "X,Y", "R,Theta"]] -> w327
                frame 0, Default {
                }
                frame 1 {
                }
                frame 2 {
                }
              }
              n52 = Equal To 0?(x="Measuring mode 3") -> (x = 0?=w332:bool)
              n53 = case shown="2" "Input ports 3" {
                tunnel: [string[] [] ("Array") string[] ["Sine out freq", "Sine out amp"] ("Array") string[] ["AUX OUT 1", "AUX OUT 2", "AUX OUT 3", "AUX OUT 4"] ("Array") string[] ["Sine out freq", "Sine out amp", "AUX OUT 1", "AUX OUT 2"] ("Array")] -> w335
                frame 0, Default {
                }
                frame 1 {
                }
                frame 2 {
                }
                frame 3 {
                }
              }
              n54 = Bundle By Name(cluster=w339, "VISA Address"="VISA resource name lock in 3", "Boolean 1"=w332, "Boolean 2"=TRUE, "String 1"="100.0_10.0", "String 2"="0.0") -> (w337:T3)
            }
          }
        }
        frame 24 {
          n55 = case shown="True" "Use Lock in 4" {
            tunnel: w355 -> [w359 w370]
            tunnel: [w359 w370] -> w351
            tunnel: [string[] [] w360] -> w352
            tunnel: [string[] [] w369] -> w353
            tunnel: w354 -> [w358 w372]
            tunnel: [w358 w371] -> w349
            frame False {
            }
            frame True {
              n56 = case shown="0, Default" "Output ports 4" {
                tunnel: [string[] ["X", "Y", "R", "Theta", "X,Y", "R,Theta", "X,Y,R,Theta", "Sensitivity"] string[] ["AUX IN 1", "AUX IN 2", "AUX IN 3", "AUX IN 4"] string[] ["X", "Y", "R", "Theta", "AUX IIN 1", "AUX IN 2", "Sensitivity", "X,Y", "R,Theta"]] -> w360
                frame 0, Default {
                }
                frame 1 {
                }
                frame 2 {
                }
              }
              n57 = Equal To 0?(x="Measuring mode 4") -> (x = 0?=w368:bool)
              n58 = case shown="2" "Input ports 4" {
                tunnel: [string[] [] ("Array") string[] ["Sine out freq", "Sine out amp"] ("Array") string[] ["AUX OUT 1", "AUX OUT 2", "AUX OUT 3", "AUX OUT 4"] ("Array") string[] ["Sine out freq", "Sine out amp", "AUX OUT 1", "AUX OUT 2"] ("Array")] -> w369
                frame 0, Default {
                }
                frame 1 {
                }
                frame 2 {
                }
                frame 3 {
                }
              }
              n59 = Bundle By Name(cluster=w372, "VISA Address"="VISA resource name lock in 4", "Boolean 1"=w368, "Boolean 2"=TRUE, "String 1"="100.0_10.0", "String 2"="0.0") -> (w371:T3)
            }
          }
        }
        frame 7 {
          n60 = case shown="False" "Use Lakeshore?" {
            tunnel: [string[] [] string[] ["Temp A", "Temp B"]] -> w380
            tunnel: w388 -> [w391 w396]
            tunnel: [w391 w394] -> w384
            tunnel: [w390 w393] -> w386
            tunnel: w387 -> [w390 w393]
            frame False {
            }
            frame True {
              n61 = Bundle By Name(cluster=w396, "VISA Address"="Lakeshore temperature controller GPIB address") -> (w394:T3)
            }
          }
        }
        frame 21 {
          n62 = case shown="True" "Use ITC He3?" {
            tunnel: [string[] [] string[] ["Temp"]] -> w397
            tunnel: w405 -> [w408 w416]
            tunnel: [w408 w415] -> w401
            tunnel: [w407 w410] -> w403
            tunnel: w404 -> [w407 w409]
            frame False {
            }
            frame True {
              n63 = call "OxITC503 _VISA_ Initialise.vi"("error in (no error)"=w409, "VISA session"="VISA Address") -> ("error out"=w410:errorcluster, "VISA session"=w411:refnum<visa-resource-name>)  [unwired: 2 in]
              n64 = Bundle By Name(cluster=w416, "VISA Address"=w411, "Int 1"="Read Item") -> (w415:T3)
            }
          }
        }
        frame 26 {
          n65 = case shown="True" "Use AH2700A?" {
            tunnel: [string[] [] string[] ["C", "Loss", "Freq", "V", "C,Loss", "C,Loss,Freq,V"]] -> w417
            tunnel: w425 -> [w428 w434]
            tunnel: [w428 w432] -> w421
            tunnel: [w427 w430] -> w423
            tunnel: w424 -> [w427 w431]
            frame False {
            }
            frame True {
              n66 = Bundle By Name(cluster=w434, "VISA Address"="VISA Address 2") -> (w433:T3)
              n67 = case shown="False" "Initialize AH2700A?" {
                tunnel: w433 -> [w438 w442]
                tunnel: [w438 w441] -> w432
                tunnel: w431 -> [w437 w440]
                tunnel: [w437 w439] -> w430
                frame False {
                }
                frame True {
                  n68 = call "Settings AH2700A (SubVI).vi"("error in"=w440, "Instrument parameters (in)"=w442) -> ("error out"=w439:errorcluster, "Instrument parameters (out)"=w441:T3)  [unwired: 8 in]
                }
              }
            }
          }
        }
        frame 8 {
          n69 = case shown="True" "Use  GPIB Write 1?" {
            tunnel: [string[] [] w462] -> w447
            tunnel: [w454 w460] -> w448
            tunnel: w451 -> [w454 w461]
            tunnel: w450 -> [w453 w458]
            tunnel: [w453 w456] -> w445
            frame False {
            }
            frame True {
              n70 = Build Array("Write") -> (w462:string[])
              n71 = case shown="True" "TEST GW1" {
                tunnel: "GW1 String 1" -> [_ w469]
                tunnel: "VISA resource name GW1" -> [_ w468]
                tunnel: w461 -> [w464 w467]
                tunnel: [w464 w466] -> w460
                frame False {
                }
                frame True {
                  n72 = call "Prompt User for Input"("Enable"=TRUE) -> ("Value"=w470:dbl)  [unwired: 16 in, 2 out]
                  n73 = call "S2DS_GW (SubVI).vi"("Value to write"=w470, "error in (no error)"=w467, "GW1 Command format"=w469, "VISA Refnum in"=w468) -> ("error out"=w466:errorcluster)  [unwired: 7 in]
                }
              }
              n74 = Bundle By Name(cluster=w458, "VISA Address"="VISA resource name GW1", "String 1"="GW1 String 1") -> (w456:T3)
            }
          }
        }
        frame 9 {
          n75 = case shown="False" "Use  GPIB Write 2?" {
            tunnel: [string[] [] w490] -> w475
            tunnel: [w482 w488] -> w476
            tunnel: w479 -> [w482 w489]
            tunnel: w478 -> [w481 w486]
            tunnel: [w481 w484] -> w473
            frame False {
            }
            frame True {
              n76 = Build Array("Write") -> (w490:string[])
              n77 = case shown="True" "TEST GW1 2" {
                tunnel: "GW2 String 1" -> [_ w495]
                tunnel: "VISA resource name GW2" -> [_ w497]
                tunnel: w489 -> [w492 w494]
                tunnel: [w492 w493] -> w488
                frame False {
                }
                frame True {
                  n78 = call "Prompt User for Input2"("Enable"=TRUE) -> ("Value"=w496:dbl)  [unwired: 16 in, 2 out]
                  n79 = Number To Exponential String(number=w496) -> ()  [unwired: 3 in, 1 out]
                  n80 = call "S2DS_GW (SubVI).vi"("Value to write"=w496, "error in (no error)"=w494, "GW1 Command format"=w495, "VISA Refnum in"=w497) -> ("error out"=w493:errorcluster)  [unwired: 7 in]
                }
              }
              n81 = Bundle By Name(cluster=w486, "VISA Address"="VISA resource name GW2", "String 1"="GW2 String 1") -> (w484:T3)
            }
          }
        }
        frame 10 {
          n82 = case shown="False" "Use  GPIB Write 3?" {
            tunnel: [string[] [] w518] -> w503
            tunnel: [w510 w516] -> w504
            tunnel: w507 -> [w510 w517]
            tunnel: w506 -> [w509 w514]
            tunnel: [w509 w512] -> w501
            frame False {
            }
            frame True {
              n83 = Build Array("Write") -> (w518:string[])
              n84 = case shown="True" "TEST GW1 3" {
                tunnel: "GW3 String 1" -> [_ w521]
                tunnel: "VISA resource name GW3" -> [_ w522]
                tunnel: w517 -> [w520 w523]
                tunnel: [w520 w524] -> w516
                frame False {
                }
                frame True {
                  n85 = call "Prompt User for Input3"("Enable"=TRUE) -> ("Value"=w525:dbl)  [unwired: 16 in, 2 out]
                  n86 = call "S2DS_GW (SubVI).vi"("Value to write"=w525, "error in (no error)"=w523, "GW1 Command format"=w521, "VISA Refnum in"=w522) -> ("error out"=w524:errorcluster)  [unwired: 7 in]
                }
              }
              n87 = Bundle By Name(cluster=w514, "VISA Address"="VISA resource name GW3", "String 1"="GW3 String 1") -> (w512:T3)
            }
          }
        }
        frame 11 {
          n88 = case shown="True" "Use  GPIB Write 4?" {
            tunnel: [string[] [] w540] -> w532
            tunnel: [w538 w545] -> w533
            tunnel: w535 -> [w538 w546]
            tunnel: w534 -> [w537 w543]
            tunnel: [w537 w539] -> w529
            frame False {
            }
            frame True {
              n89 = Build Array("Write") -> (w540:string[])
              n90 = case shown="True" "TEST GW4" {
                tunnel: "GW4 String 2" -> [_ w549]
                tunnel: "VISA resource name GW4" -> [_ w552]
                tunnel: w546 -> [w548 w550]
                tunnel: [w548 w551] -> w545
                frame False {
                }
                frame True {
                  n91 = call "Prompt User for Input4"("Enable"=TRUE) -> ("Value"=w553:dbl)  [unwired: 16 in, 2 out]
                  n92 = call "S2DS_GW (SubVI).vi"("Value to write"=w553, "error in (no error)"=w550, "GW1 Command format"=w549, "VISA Refnum in"=w552) -> ("error out"=w551:errorcluster)  [unwired: 7 in]
                }
              }
              n93 = Bundle By Name(cluster=w543, "VISA Address"="VISA resource name GW4", "String 1"="GW4 String 2") -> (w539:T3)
            }
          }
        }
        frame 12 {
          n94 = case shown="True" "Use VISA Read 1" {
            tunnel: [string[] [] w575] -> w559
            tunnel: [w566 w569] -> w560
            tunnel: w562 -> [w566 w569]
            tunnel: w563 -> [w565 w574]
            tunnel: [w565 w573] -> w557
            frame False {
            }
            frame True {
              n95 = Build Array("Read") -> (w575:string[])
              n96 = Unbundle By Name("Visa Read") -> ("VISA resource"=w567:refnum<visa-resource-name>, "Read Command"=w572:string, "Format string"=w571:string)
              n97 = case shown="True" "TEST GR1" {
                tunnel: w567 -> [_ w579]
                tunnel: w572 -> [_ w578]
                tunnel: w571 -> [_ w577]
                frame False {
                }
                frame True {
                  n98 = call "S2DS_GR-test.vi"("Write command"=w578, "format string"=w577, "VISA Refnum in"=w579) -> ()  [unwired: 6 in, 3 out]
                }
              }
              n99 = Bundle By Name(cluster=w574, "VISA Address"=w567, "String 1"=w572, "String 2"=w571) -> (w573:T3)
            }
          }
        }
        frame 13 {
          n100 = case shown="True" "Use VISA Read 2" {
            tunnel: [string[] [] w600] -> w584
            tunnel: [w591 w593] -> w585
            tunnel: w587 -> [w591 w593]
            tunnel: w588 -> [w590 w599]
            tunnel: [w590 w598] -> w582
            frame False {
            }
            frame True {
              n101 = Build Array("Read") -> (w600:string[])
              n102 = Unbundle By Name("Visa Read 2") -> ("VISA resource"=w592:refnum<visa-resource-name>, "Read Command"=w597:string, "Format string"=w596:string)
              n103 = case shown="True" "TEST GR1 2" {
                tunnel: w592 -> [_ w604]
                tunnel: w597 -> [_ w603]
                tunnel: w596 -> [_ w602]
                frame False {
                }
                frame True {
                  n104 = call "S2DS_GR-test.vi"("Write command"=w603, "format string"=w602, "VISA Refnum in"=w604) -> ()  [unwired: 6 in, 3 out]
                }
              }
              n105 = Bundle By Name(cluster=w599, "VISA Address"=w592, "String 1"=w597, "String 2"=w596) -> (w598:T3)
            }
          }
        }
        frame 14 {
          n106 = case shown="True" "Use VISA Read 3" {
            tunnel: [string[] [] w625] -> w609
            tunnel: [w616 w619] -> w610
            tunnel: w612 -> [w616 w619]
            tunnel: w613 -> [w615 w624]
            tunnel: [w615 w623] -> w607
            frame False {
            }
            frame True {
              n107 = Build Array("Read") -> (w625:string[])
              n108 = Unbundle By Name("Visa Read 3") -> ("VISA resource"=w618:refnum<visa-resource-name>, "Read Command"=w622:string, "Format string"=w621:string)
              n109 = case shown="True" "TEST GR1 3" {
                tunnel: w618 -> [_ w629]
                tunnel: w622 -> [_ w628]
                tunnel: w621 -> [_ w627]
                frame False {
                }
                frame True {
                  n110 = call "S2DS_GR-test.vi"("Write command"=w628, "format string"=w627, "VISA Refnum in"=w629) -> ()  [unwired: 6 in, 3 out]
                }
              }
              n111 = Bundle By Name(cluster=w624, "VISA Address"=w618, "String 1"=w622, "String 2"=w621) -> (w623:T3)
            }
          }
        }
        frame 15 {
          n112 = case shown="True" "Use VISA Read 4" {
            tunnel: [string[] [] w650] -> w634
            tunnel: [w641 w643] -> w635
            tunnel: w637 -> [w641 w643]
            tunnel: w638 -> [w640 w649]
            tunnel: [w640 w648] -> w632
            frame False {
            }
            frame True {
              n113 = Build Array("Read") -> (w650:string[])
              n114 = Unbundle By Name("Visa Read 4") -> ("VISA resource"=w644:refnum<visa-resource-name>, "Read Command"=w647:string, "Format string"=w646:string)
              n115 = case shown="True" "TEST GR1 4" {
                tunnel: w644 -> [_ w654]
                tunnel: w647 -> [_ w653]
                tunnel: w646 -> [_ w652]
                frame False {
                }
                frame True {
                  n116 = call "S2DS_GR-test.vi"("Write command"=w653, "format string"=w652, "VISA Refnum in"=w654) -> ()  [unwired: 6 in, 3 out]
                }
              }
              n117 = Bundle By Name(cluster=w649, "VISA Address"=w644, "String 1"=w647, "String 2"=w646) -> (w648:T3)
            }
          }
        }
        frame 16 {
          n118 = case shown="True" "Use SMU?" {
            tunnel: [string[] [] w679] -> w660
            tunnel: [string[] [] w678] -> w659
            tunnel: [w667 w671] -> w661
            tunnel: w663 -> [w667 w670]
            tunnel: [T10 {"VISA Address"="", "GPIB/TCP Address"="", "String 1"="", "String 2"="", "Boolean 1"=FALSE, "Boolean 2"=FALSE, "Integer 1"=0, "Integer 2"=0, "Double 1"=0.0, "Double 2"=0.0} ("output cluster") w682] -> w657
            tunnel: w662 -> [_ w677]
            frame False {
            }
            frame True {
              w680 = "Sourcemeter"
              n119 = Build Array(w680) -> (w678:string[])
              n120 = Build Array(w680) -> (w679:string[])
              n121 = call "Initialize Sourcemeter (Pratap).vi"("Source Value"="Source Value", "Compliance Limit"="Compliance Limit", "error in (no error)"=w670, "Reset (True)"="Resset SMU?", "Source Function"="Source", "VISA Refnum in"="SMU VISA Address") -> ("error out"=w671:errorcluster, "Node Out"=w672:string, "VISA Refnum out"=w673:refnum<visa-resource-name>)  [unwired: 3 in]
              n122 = Bundle By Name(cluster=w677, "VISA Address"=w673, "String 1"=w672, "Int 1"="Source", "Int 2"="Measure") -> (w682:T3)
            }
          }
        }
        frame 17 {
          n123 = case shown="True" "Use DS360 Func Gen?" {
            tunnel: [string[] [] string[] ["frequency", "amplitude", "offset"]] -> w684
            tunnel: [w694 w699] -> w688
            tunnel: w690 -> [w694 w699]
            tunnel: w691 -> [w693 w698]
            tunnel: [w693 w697] -> w687
            frame False {
            }
            frame True {
              n124 = Bundle By Name(cluster=w698, "GPIB/TCP Address"="DS360 Function Generator GPIB address") -> (w697:T3)
            }
          }
        }
        frame 18 {
          n125 = case shown="True" "Use Current source?" {
            tunnel: [string[] [] string[] ["current"]] -> w701
            tunnel: [w711 w717] -> w705
            tunnel: w707 -> [w711 w718]
            tunnel: w708 -> [w710 w722]
            tunnel: [w710 w721] -> w704
            frame False {
            }
            frame True {
              n126 = call "My Current source Initialization (SubVI).vi"("Output Low Connection"="Output Low \nConnection", "Current level"="Current level", "error in (no error)"=w718, "Current Range In"="Current Range In", "Voltage limit (V)"="Voltage limit (V)", "VISA Refnum in"="Current source VISA Address") -> ("error out"=w717:errorcluster, "VISA Refnum out"=w719:refnum<visa-resource-name>)  [unwired: 4 in]
              n127 = Bundle By Name(cluster=w722, "Double 1"="Voltage limit (V)", "VISA Address"=w719) -> (w721:T3)
            }
          }
        }
        frame 25 {
          n128 = case shown="True" "Use Keithley 2182 Nanovoltmeter?" {
            tunnel: [string[] [] string[] []] -> w725
            tunnel: [w735 w736] -> w728
            tunnel: w730 -> [w735 w737]
            tunnel: w731 -> [w734 w744]
            tunnel: [w734 w741] -> w727
            tunnel: [string[] [] ("RC names") string[] ["Voltage"] ("RC names")] -> w723
            frame False {
            }
            frame True {
              n129 = Bundle By Name(cluster=w744, "VISA Address"="Keithley 2182 address") -> (w740:T3)
              n130 = case shown="True" "Resset SMU? 2" {
                tunnel: [w746 w749] -> w741
                tunnel: w740 -> [w746 w750]
                tunnel: w737 -> [w745 w748]
                tunnel: [w745 w747] -> w736
                frame False {
                }
                frame True {
                  n131 = call "Keithley 2182 Edit Settings.vi"("error in"=w748, "Instrument parameters in"=w750) -> ("error out"=w747:errorcluster, "Instrument parameters out"=w749:T10)  [unwired: 8 in]
                }
              }
            }
          }
        }
        frame 19 {
          n132 = case shown="True" "Use External 1?" {
            tunnel: [w760 w766] -> w753
            tunnel: [w762 w764] -> w756
            tunnel: w758 -> [w762 w765]
            tunnel: w759 -> [w761 w770]
            tunnel: [w761 w767] -> w755
            tunnel: [w760 w763] -> w751
            frame False {
              w760 = string[] []
            }
            frame True {
              n133 = call "S2DS_Open dstp for external write (SubVI).vi"("error in (no error)"=w765, "Number identifier"=1 ("Numeric"), "External Write instrument settings"="?", "Instrument parameters in"=w770) -> ("error out"=w764:errorcluster, "Read port list"=w763:string[], "Write port list"=w766:string[], "Instrument parameters out"=w767:T3)  [unwired: 4 in]
            }
          }
        }
        frame 20 {
          n134 = case shown="False" "Use External 2?" {
            tunnel: [w780 w786] -> w773
            tunnel: [w782 w784] -> w776
            tunnel: w778 -> [w782 w785]
            tunnel: w779 -> [w781 w790]
            tunnel: [w781 w787] -> w775
            tunnel: [w780 w783] -> w771
            frame False {
              w780 = string[] []
            }
            frame True {
              n135 = call "S2DS_Open dstp for external write (SubVI).vi"("error in (no error)"=w785, "Number identifier"=2 ("Numeric"), "External Write instrument settings"="?", "Instrument parameters in"=w790) -> ("error out"=w784:errorcluster, "Read port list"=w783:string[], "Write port list"=w786:string[], "Instrument parameters out"=w787:T3)  [unwired: 4 in]
            }
          }
        }
        frame 22 {
          n136 = case shown="True" w791 {
            tunnel: [w800 string[] []] -> w793
            tunnel: [w802 w810] -> w796
            tunnel: w798 -> [w802 w810]
            tunnel: w799 -> [w801 w806]
            tunnel: [w801 w805] -> w795
            tunnel: [w800 string[] []] -> w792
            frame False {
              w800 = string[] []
            }
            frame True {
              n137 = Bundle By Name(cluster=w806, "GPIB/TCP Address"="dstp://localhost/S2DSIndex" ("Write Location"), "String 1"="dstp://localhost/ArrayIndex" ("Write Location"), "String 2"="dstp://localhost/ArrayData" ("Write Location")) -> (w805:T3)
            }
          }
        }
        frame 29, Default {
          w813 = string[] [] ("RC names")
        }
      }
      n138 = case shown="True" w67 {
        tunnel: w57 -> [_ w81]
        tunnel: w59 -> [_ w73]
        tunnel: [w72 w78] -> w65
        tunnel: w66 -> [w72 w80]
        tunnel: w56 -> [_ w77]
        tunnel: [w71 w74] -> w63
        tunnel: w64 -> [w71 w75]
        frame False {
        }
        frame True {
          n139 = for {
            tunnel: w81 -> [w87] mode=indexing
            tunnel: w73 -> [w89]
            tunnel: [w86] -> w79 mode=indexing
            n140 = Concatenate Strings(w89, ":" ("string"), w87) -> (w86:string)
          }
          n141 = for {
            tunnel: w77 -> [w83] mode=indexing
            tunnel: w73 -> [w85]
            tunnel: [w82] -> w76 mode=indexing
            n142 = Concatenate Strings(w85, ":" ("string"), w83) -> (w82:string)
          }
          n143 = Build Array (concatenate)(w80, w79) -> (w78:string[])
          n144 = Build Array (concatenate)(w75, w76) -> (w74:string[])
        }
      }
      "Use array instrument" <- "Use array instrument"
    }
    "Error status:" <- w43
    n145 = Index Array(array=w34, index=w33) -> (element=w35:T3)
    n146 = Build Array (concatenate)(w37, w35) -> (w36:T3[])
    n147 = case shown="True" "Clear error" {
      tunnel: [w53 errorcluster {"status"=FALSE, "code"=0, "source"=""} ("error in")] -> w40
      tunnel: w43 -> [w53 _]
      frame False {
      }
      frame True {
      }
    }
  }
  "Error (out)" <- w16
  "OK 2" <- w4
  n148 = Unbundle By Name("Port list (in)") -> ("Write ports"=w20:string[], "Read ports"=w21:string[])
  n149 = Unbundle By Name("Instrument Info (in)") -> ("Instrument parameters"=w10:T3[], "Total Instrument List"=w2:string[])
  n150 = for {
    tunnel: w12 -> [w823] mode=indexing
    tunnel: w3 -> [w822] mode=indexing
    tunnel: w11 -> [w821] mode=indexing
    shift-right: [w819] -> w9
    shift-left: w10 -> [w820]
    shift-right: [w817] -> w8
    shift-left: w2 -> [w818]
    n151 = case shown="True" w823 {
      tunnel: w822 -> [_ w831]
      tunnel: w821 -> [_ w830]
      tunnel: w820 -> [w825 w829]
      tunnel: [w825 w828] -> w819
      tunnel: w818 -> [w824 w827]
      tunnel: [w824 w826] -> w817
      frame False {
      }
      frame True {
        n152 = Build Array (concatenate)(w829, w830) -> (w828:T3[])
        n153 = Build Array (concatenate)(w827, w831) -> (w826:string[])
      }
    }
  }
  n154 = Build Array (concatenate)(w20, w29, "None") -> (w26:string[])
  n155 = Build Array (concatenate)(w21, "Random", w31, "Time", "None") -> (w25:string[])
  n156 = Bundle By Name(cluster="Port list (in)", "Write ports"=w26, "Read ports"=w25) -> (→"Port lists (out)":T1)
  n157 = Build Array (concatenate)(w2) -> (w1:string[])
  n158 = Bundle By Name(cluster="Instrument Info (in)", "Instrument parameters"=w9, "DAQ Tasks"=w23, "Total Instrument List"=w8, "User instrument list"=w1) -> (→"Instrument info (out)":T2)
